vi "Create.vi"(8 "error in (no error)":errorcluster, 10 "flow rate":dbl, 11 "obj":refnum<class "SimPump.lvclass">) -> (0 "error out":errorcluster, 3 "obj out":refnum<class "SimPump.lvclass">)   [LabVIEW 2019, in "SimPump.lvclass"]
doc: "Creates a bike object\n\nwww.sciware.com.au"
uses:
  SimPump.lvclass
  Private/DataMembers.ctl
  SimPump.lvclass/SimPump.ctl
panel:
  in  "data members (type)":T1
  # "BSD License (http://www.opensource.org/licenses/bsd-license.php)"
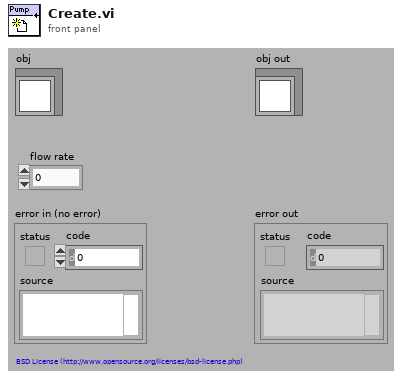
[diagram p1: front panel]
types:
  T1 = typedef "SimPump.lvclass/DataMembers.ctl" = cluster{"flow rate":dbl, "volume to pump":dbl, "state":bool, "ti":u32, "t0":u32}
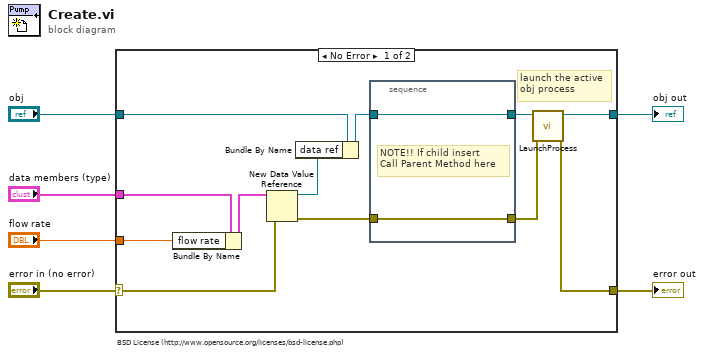
[diagram p0: block diagram]
diagram:
  # "BSD License (http://www.opensource.org/licenses/bsd-license.php)"
  n1 = case shown="No Error" "error in (no error)" {
    selector: "error in (no error)" -> [w18 w22]
    tunnel: [w16 w22] -> w5
    tunnel: "data members (type)" -> [w9 _]
    tunnel: [w15 w21] -> w3
    tunnel: "obj" -> [w14 w21]
    tunnel: "flow rate" -> [w7 _]
    frame No Error {
      # "launch the active\nobj process"
      n2 = Bundle By Name(cluster=w9, "flow rate"=w7) -> (w8:T1)
      n3 = New Data Value Reference(data value=w8, error in=w18) -> (data value reference=w17:refnum<data-value>, error out=w11:errorcluster)
      n4 = Bundle By Name(cluster=w14, "data ref"=w17) -> (w13:refnum<class "SimPump.lvclass">)
      n5 = stacked-sequence {
        tunnel: [w20] -> w12
        tunnel: w13 -> [w20]
        tunnel: w11 -> [w19]
        tunnel: [w19] -> w10
        frame #0 {
          # "NOTE!! If child insert\nCall Parent Method here"
        }
      }
      n6 = call-dynamic "LaunchProcess.vi"("error in (no error)"=w10, "obj"=w12) -> ("error out"=w16:errorcluster, "obj out"=w15:refnum<class "SimPump.lvclass">)  [unwired: 8 in]
    }
    frame Error {
    }
  }
  "error out" <- w5
  "obj out" <- w3
